vi "Write configuration.vi"(8 "error in (no error)":errorcluster, 11 "BMC in":refnum<class "BMC.lvclass">) -> (0 "error out":errorcluster, 3 "BMC out":refnum<class "BMC.lvclass">)   [LabVIEW 2012, in "BMC.lvclass"]
doc: "Writes the configuration cluster into the configuration file. Configuration file is XML-based. It's name is <component ID>.xml"
uses:
  BMC.lvclass
  Murmex/LabVIEW/Murmex/Murmex/Murmex.lvclass
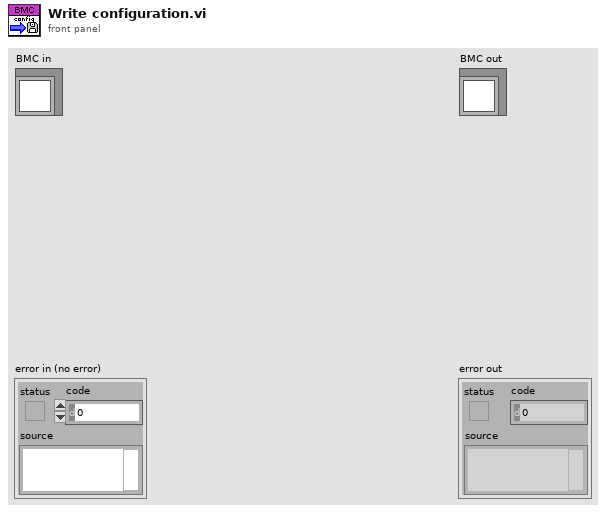
[diagram p1: front panel]
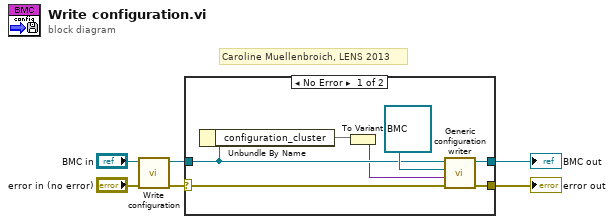
[diagram p0: block diagram]
diagram:
  # "Caroline Muellenbroich, LENS 2013"
  n1 = call-parent "Write configuration.vi"("error in (no error)"="error in (no error)", "Murmex in"="BMC in") -> ("error out"=w4:errorcluster, "Murmex out"=w1:refnum<class "BMC.lvclass">)  [unwired: 8 in]
  n2 = case shown="No Error" w4 {
    selector: w4 -> [w11 w15]
    tunnel: [w10 w15] -> w3
    tunnel: [w12 w14] -> w2
    tunnel: w1 -> [w9 w14]
    frame No Error {
      n3 = Unbundle By Name(w9) -> ("configuration_cluster"=w8)
      n4 = To Variant(anything=w8) -> (Variant=w7:variant)
      n5 = call "Generic configuration writer.vi"("error in (no error)"=w11, "configuration"=w7, "inheritance level"=refnum<class "BMC.lvclass"> refnum ("BMC"), "MurmexBase in"=w9) -> ("error out"=w10:errorcluster, "MurmexBase out"=w12:refnum<class "BMC.lvclass">)  [unwired: 6 in]
    }
    frame Error {
    }
  }
  "error out" <- w3
  "BMC out" <- w2
